vi "Voltages_2_I16.vi"(1 "Voltages":dbl[](array[numeric]), 2 "Av Sampling Rate":dbl) -> (0 "Channel Data":T1)   [LabVIEW 2017]
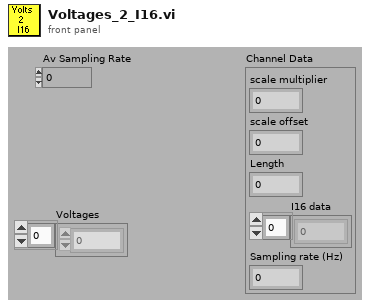
[diagram p1: front panel]
types:
  T1 = cluster{"scale multiplier":dbl, "scale offset":dbl, "Length":i32, "I16 data":i16[], "Sampling rate (Hz)":dbl}
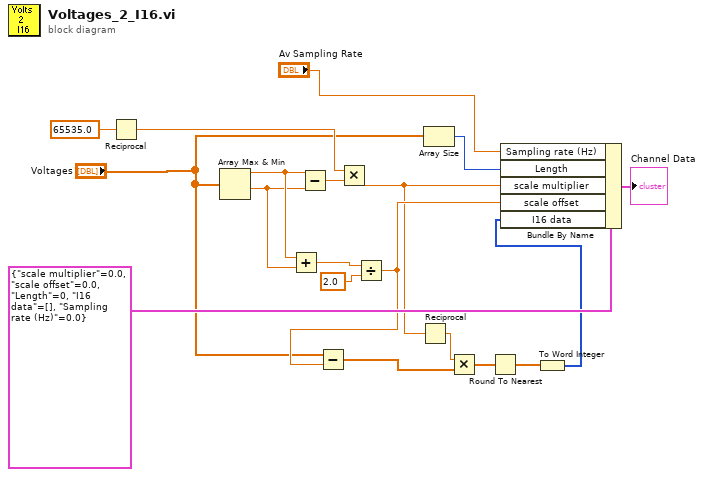
[diagram p0: block diagram]
diagram:
  n1 = Reciprocal(x=65535.0 ("y")) -> (1/x=w18:dbl)
  n2 = Array Max & Min(array="Voltages") -> (max value=w16:dbl, min value=w15:dbl)  [unwired: 2 out]
  n3 = Add(x=w16, y=w15) -> (x+y=w14:dbl)
  n4 = Subtract(x=w16, y=w15) -> (x-y=w10:dbl)
  n5 = Multiply(x=w18, y=w10) -> (x*y=w9:dbl)
  n6 = Divide(x=w14, y=2.0) -> (x/y=w12:dbl)
  n7 = Subtract(x="Voltages", y=w12) -> (x-y=w7:dbl[])
  n8 = Reciprocal(x=w9) -> (1/x=w8:dbl)
  n9 = Array Size(array="Voltages") -> (size(s)=w4:i32)
  n10 = Multiply(x=w8, y=w7) -> (x*y=w6:dbl[])
  n11 = Round To Nearest(number=w6) -> (nearest integer value=w11:dbl[])
  n12 = To Word Integer(number=w11) -> (16bit integer=w3:i16[])
  n13 = Bundle By Name(cluster=T1 {"scale multiplier"=0.0, "scale offset"=0.0, "Length"=0, "I16 data"=[], "Sampling rate (Hz)"=0.0}, "Sampling rate (Hz)"="Av Sampling Rate", "Length"=w4, "scale multiplier"=w9, "scale offset"=w12, "I16 data"=w3) -> (→"Channel Data":T1)
